vi "Display Two Button Popup (Plain).vi"(4 "keep transparent buttons?":bool=TRUE, 5 "N-Text":string="No", 6 "Theme":refnum<class "Theme.lvclass">, 7 "Y-Text":string="Yes", 8 "error in":errorcluster, 10 "Message":string, 11 "Dialog Title":string) -> (0 "error out":errorcluster, 1 "Choice":bool)   [LabVIEW 2021, in "Pop-Up.lvlib" / "Plain - Two Button.lvclass"]
doc: "The two button popup will display information to the user and wait for the operator to click the button to make a choice.\n\n<b>Note:</b> The function <b>Close Pop-Up.vi</b> can be used to close this dialog early.\n\n<b>Note:</b> The dialog vertical sizing will adjust for longer messages, so <b>test</b> all messages prior to deployment to make sure that scaling fits.\n\nInputs: +\n-Dialog Title [String] - String variable to populate the dialog's title bar +\n-Message [String] - String Variable to populate Display +\n-Theme [lvclass] - the theme for the style of the popup +\n-Y-Text [String] - the button text for the <b>yes</b> button (right) +\n-N-Text [String] - the button text for the <b>no</b> button (left) +\n-Keep transparent buttons? [Boolean] - choose to leave buttons transparent (T) or use theme colors (F)\n\nOutputs: +\n-Choice [Boolean] - true/false of user selection\n\n<b>Code Developed By:</b> +\nDaniel Coons +\nhttps://github.com/danielcoons/tsc-pop-up"
uses:
  Plain - Two Button.lvclass
  Theme/Theme.lvclass
  C:/Development/Open Source/tsc-pop-up/Popup/Popup.lvclass
  C:/Development/Open Source/tsc-pop-up/Plain/Plain Parent.lvclass
  Plain Parent.lvclass/Plain Parent.ctl
  Write Dialog Title.vi
  Write Action 1 Text.vi
  Write Action 2 Text.vi
  Set Transparent buttons.vi
  Popup/Data Member Access/Write Theme.vi
  Plain - Two Button.lvclass/Plain - Two Button.ctl
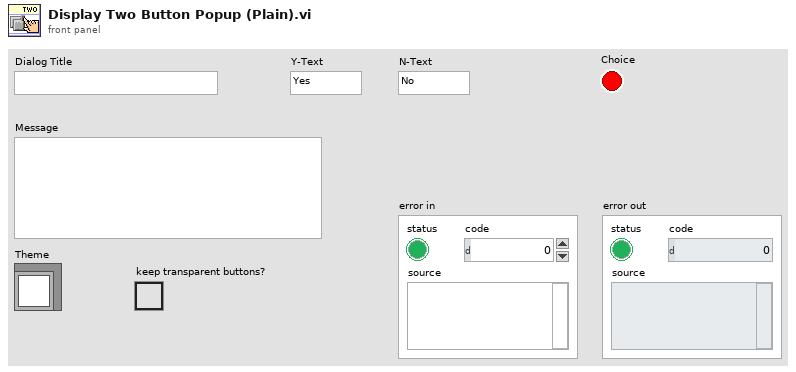
[diagram p1: front panel]
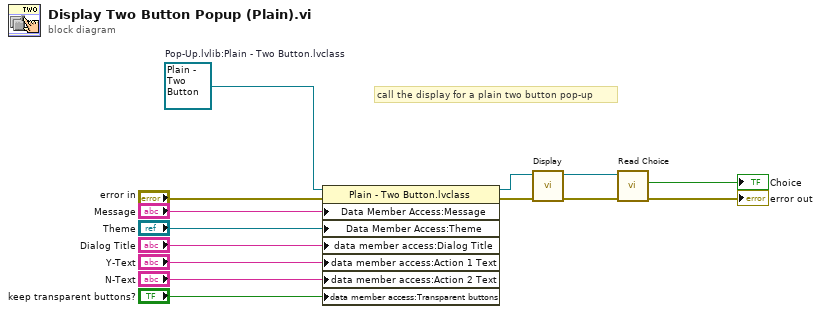
[diagram p0: block diagram]
diagram:
  w2 = refnum<class "Plain - Two Button.lvclass"> refnum  # Pop-Up.lvlib:Plain - Two Button.lvclass
  # "call the display for a plain two button pop-up"
  n1 = property class="Plain - Two Button.lvclass"(reference=w2, error in="error in", "Data Member Access:Message"="Message", "Data Member Access:Theme"="Theme", "data member access:Dialog Title"="Dialog Title", "data member access:Action 1 Text"="Y-Text", "data member access:Action 2 Text"="N-Text", "data member access:Transparent buttons"="keep transparent buttons?") -> (reference out=w11:refnum<class "Plain - Two Button.lvclass">, error out=w12:errorcluster)
  n2 = call-dynamic "Display.vi"("error in"=w12, "Plain - Two Button in"=w11) -> ("error out"=w14:errorcluster, "Plain - Two Button out"=w4:refnum<class "Plain - Two Button.lvclass">)  [unwired: 8 in]
  n3 = call-dynamic "Read Choice.vi"("error in (no error)"=w14, "_Popup in"=w4) -> ("error out"=→"error out":errorcluster, "Choice"=→"Choice":bool)  [unwired: 7 in, 1 out]
